vi "_Auto Analysis.vi"(8 "error in (no error)":errorcluster, 11 "Yokogawa AQ6370D in":refnum<class "Yokogawa AQ6370D.lvclass">) -> (0 "error out":errorcluster, 2 "Analysis Data":T1, 3 "Yokogawa AQ6370D out":refnum<class "Yokogawa AQ6370D.lvclass">)   [LabVIEW 2018, in "Yokogawa AQ6370D.lvlib" / "Yokogawa AQ6370D.lvclass"]
uses:
  Yokogawa AQ6370D.lvclass
  Parent/Custom Controls/Analysis Data.ctl
  Yokogawa AQ6370D.lvclass/Yokogawa AQ6370D.ctl
  builds/OSA.lvlibp/Optical Spectrum Analyzer.lvclass
  Parent/Optical Spectrum Analyzer.lvclass
  C:/Projects/LabVIEW/In-Progress/Chetan Malpure/Optical Spectrum Analyzer/builds/OSA.lvlibp/Optical Spectrum Analyzer.lvclass
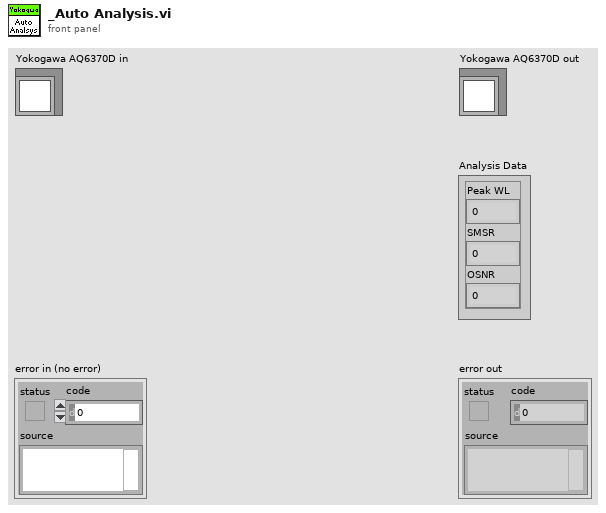
[diagram p1: front panel]
types:
  T1 = typedef "Optical Spectrum Analyzer.lvlib/Optical Spectrum Analyzer.lvclass/Analysis Data.ctl" = cluster{"Peak WL":dbl, "SMSR":dbl, "OSNR":dbl}
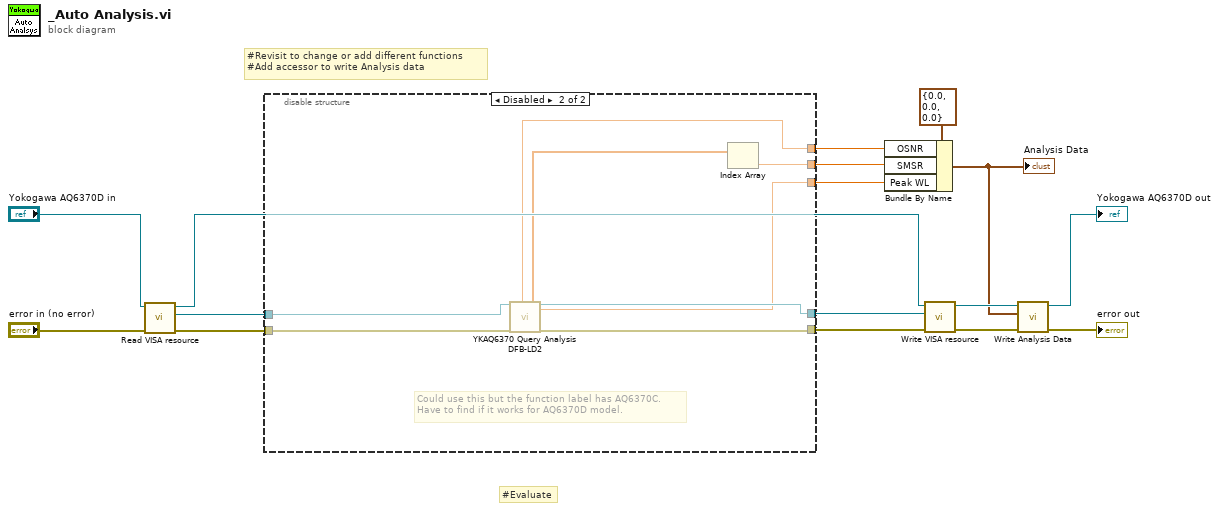
[diagram p0: block diagram]
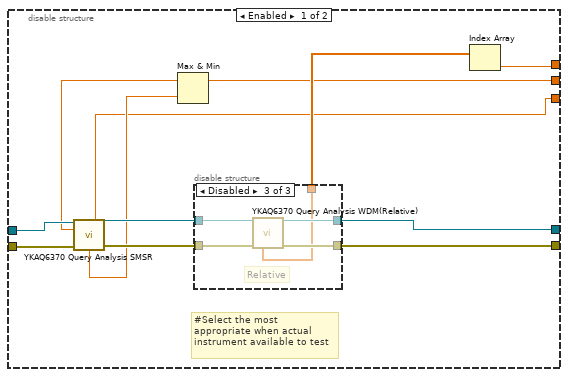
[diagram p2: hidden frame]
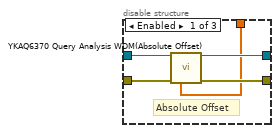
[diagram p3: hidden frame]
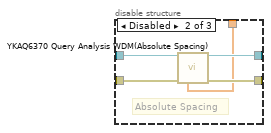
[diagram p4: hidden frame]
diagram:
  # "#Evaluate"
  # "#Revisit to change or add different functions\n#Add accessor to write Analysis data"
  n1 = call "Read VISA resource.vi"("error in (no error)"="error in (no error)", "Yokogawa AQ6370D in"="Yokogawa AQ6370D in") -> ("error out"=w15:errorcluster, "VISA resource"=w13:refnum<visa-resource-name>, "Yokogawa AQ6370D out"=w11:refnum<class "Yokogawa AQ6370D.lvclass">)  [unwired: 7 in]
  n2 = disable-structure shown="Disabled" {
    disable-tunnel: w15 -> [w28 w50]
    disable-tunnel: w13 -> [w27 w51]
    disable-tunnel: [w24 w49] -> w12
    disable-tunnel: [w23 w48] -> w10
    disable-tunnel: [w19 w44] -> w4
    disable-tunnel: [w17 w46] -> w3
    disable-tunnel: [w18 w45] -> w1
    frame Enabled {
      # "#Select the most \nappropriate when actual \ninstrument available to test"
      n3 = call <instrlib>:"YKAQ6370 Query Analysis SMSR.vi"("VISA resource name"=w27, "error in (no error)"=w28) -> ("Peak WL"=w18:dbl, "VISA resource name out"=w25:refnum<visa-resource-name>, "Delta Level(R)"=w21:dbl, "Delta Level"=w22:dbl, "error out"=w26:errorcluster)  [unwired: 2 in, 7 out]
      n4 = Max & Min(x=w21, y=w22) -> (max(x,y)=w17:dbl)  [unwired: 1 out]
      n5 = disable-structure shown="Disabled" {
        disable-tunnel: w26 -> [w33 w37 w40]
        disable-tunnel: w25 -> [w32 w38 w43]
        disable-tunnel: [w31 w35 w41] -> w24
        disable-tunnel: [w30 w36 w42] -> w23
        disable-tunnel: [w29 w34 w39] -> w20
        frame Enabled {
          # "Absolute Offset"
          n6 = call <instrlib>:"YKAQ6370 Query Analysis WDM(Absolute Offset).vi"("VISA resource name"=w32, "error in (no error)"=w33) -> ("VISA resource name out"=w30:refnum<visa-resource-name>, "SNR"=w29:dbl[], "error out"=w31:errorcluster)  [unwired: 5 in, 6 out]
        }
        frame Disabled {
          # "Absolute Spacing"
          n7 = call <instrlib>:"YKAQ6370 Query Analysis WDM(Absolute Spacing).vi"("VISA resource name"=w38, "error in (no error)"=w37) -> ("VISA resource name out"=w36:refnum<visa-resource-name>, "SNR"=w34:dbl[], "error out"=w35:errorcluster)  [unwired: 5 in, 6 out]
        }
        frame Disabled {
          # "Relative"
          n8 = call <instrlib>:"YKAQ6370 Query Analysis WDM(Relative).vi"("VISA resource name"=w43, "error in (no error)"=w40) -> ("VISA resource name out"=w42:refnum<visa-resource-name>, "SNR"=w39:dbl[], "error out"=w41:errorcluster)  [unwired: 5 in, 6 out]
        }
      }
      n9 = Index Array(array=w20) -> (element=w19:dbl)  [unwired: 1 in]
    }
    frame Disabled {
      # "Could use this but the function label has AQ6370C.\nHave to find if it works for AQ6370D model."
      n10 = call <instrlib>:"YKAQ6370 Query Analysis DFB-LD2.vi"("VISA resource name"=w51, "error in (no error)"=w50) -> ("OSNR"=w44:dbl, "SMSR"=w47:dbl[], "VISA resource name out"=w48:refnum<visa-resource-name>, "Peak WL"=w45:dbl, "error out"=w49:errorcluster)  [unwired: 6 in, 7 out]
      n11 = Index Array(array=w47) -> (element=w46:dbl)  [unwired: 1 in]
    }
  }
  n12 = Bundle By Name(cluster=T1 {"Peak WL"=0.0, "SMSR"=0.0, "OSNR"=0.0} ("Analysis Data"), "OSNR"=w4, "SMSR"=w3, "Peak WL"=w1) -> (w2:T1)
  "Analysis Data" <- w2
  n13 = call "Write VISA resource.vi"("error in (no error)"=w12, "VISA resource"=w10, "Yokogawa AQ6370D in"=w11) -> ("error out"=w8:errorcluster, "Yokogawa AQ6370D out"=w9:refnum<class "Yokogawa AQ6370D.lvclass">)  [unwired: 7 in]
  n14 = call "Write Analysis Data.vi"("error in (no error)"=w8, "Analysis Data"=w2, "Optical Spectrum Analyzer in"=w9) -> ("error out"=→"error out":errorcluster, "Optical Spectrum Analyzer out"=→"Yokogawa AQ6370D out":refnum<class "Yokogawa AQ6370D.lvclass">)  [unwired: 7 in]
